vi "WSVCAP SHL FPGA LL RFFE Read Data.vi"(11 "error in (no error)":errorcluster, 12 "Socket Mask":u16) -> (4 "Word Out (1-Bit for Each Channel)":u16, 15 "error out":errorcluster)   [LabVIEW 2012]
uses:
  WSVCAP SHL FPGA LL RFFE Debug Global.vi
  <vilib>/eio/EIONode/EIONode.xnode
  <vilib>/rvi/eio/common/nirviEmuTemplateMethod_errors.vi
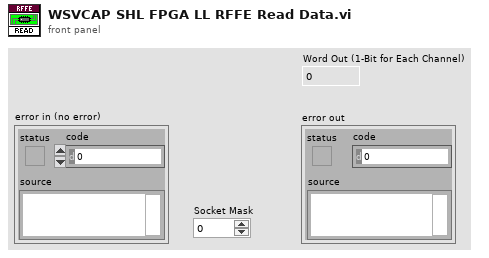
[diagram p1: front panel]
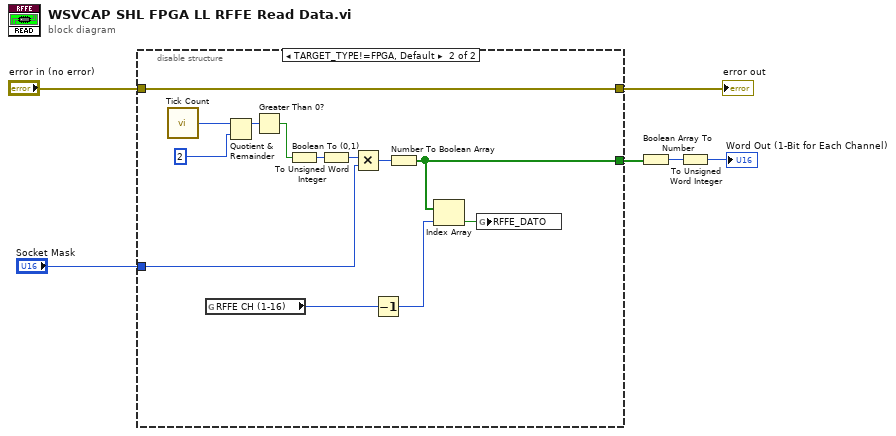
[diagram p0: block diagram]
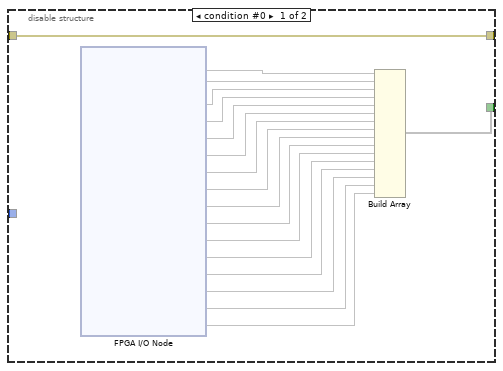
[diagram p2: hidden frame]
diagram:
  n1 = disable-structure shown="TARGET_TYPE!=FPGA, Default" {
    disable-tunnel: [w8 w27] -> w2
    disable-tunnel: [w7 w34] -> w6
    disable-tunnel: "error in (no error)" -> [w7 w34]
    disable-tunnel: "Socket Mask" -> [_ w31]
    frame condition #0 {
      n2 = xnode "FPGA I/O Node"() -> ("RFFE_DATO_S1"=w9, "RFFE_DATO_S2"=w24, "RFFE_DATO_S3"=w23, "RFFE_DATO_S4"=w22, "RFFE_DATO_S5"=w21, "RFFE_DATO_S6"=w20, "RFFE_DATO_S7"=w19, "RFFE_DATO_S8"=w18, "RFFE_DATO_S9"=w17, "RFFE_DATO_S10"=w16, "RFFE_DATO_S11"=w15, "RFFE_DATO_S12"=w14, "RFFE_DATO_S13"=w13, "RFFE_DATO_S14"=w12, "RFFE_DATO_S15"=w11, "RFFE_DATO_S16"=w10)  [unwired: 16 in, 16 out]
      n3 = Build Array(w9, w24, w23, w22, w21, w20, w19, w18, w17, w16, w15, w14, w13, w12, w11, w10) -> (w8:void[])
    }
    frame condition #1 (active) {
      n4 = call "Tick Count"() -> ("Tick Count(Ticks)"=w37:u32)
      n5 = global read "WSVCAP SHL FPGA LL RFFE Debug Global.vi" "RFFE CH (1-16)"() -> (w29:i32)
      n6 = Quotient & Remainder(x=w37, y=u32 2) -> (x-y*floor(x/y)=w36:u32)  [unwired: 1 out]
      n7 = Greater Than 0?(x=w36) -> (x > 0?=w25:bool)
      n8 = Boolean To (0,1)(Boolean=w25) -> (0, 1=w33:i16)
      n9 = To Unsigned Word Integer(number=w33) -> (unsigned 16bit integer=w32:u16)
      n10 = Multiply(x=w32, y=w31) -> (x*y=w30:u16)
      n11 = Decrement(x=w29) -> (x-1=w26:i32)
      n12 = Number To Boolean Array(number=w30) -> (Boolean array=w27:bool[])
      n13 = Index Array(array=w27, index=w26) -> (element=w28:bool)
      n14 = global write "WSVCAP SHL FPGA LL RFFE Debug Global.vi" "RFFE_DATO"(w28) -> ()
    }
  }
  "error out" <- w6
  n15 = Boolean Array To Number(Boolean array=w2) -> (number=w3:u16)
  n16 = To Unsigned Word Integer(number=w3) -> (unsigned 16bit integer=→"Word Out (1-Bit for Each Channel)":u16)
